vi "Set S34CON wrapper.vi"(7 "bAckEna":i32, 8 "error in (no error)":errorcluster caption="错误输入（无错误）", 9 "S34CON In":T1, 10 "dwCanNodeId":u32, 11 "dwDevIndex":u32) -> (0 "error out":errorcluster caption="错误输出", 1 "S34CON Out":T1, 3 "function return":u32)   [LabVIEW 2016, in "UISimCanFunc_wrapper.lvlib"]
doc: "_declspec (dllexport) DWORD SetS34CON_wrapper(DWORD dwDevIndex, DWORD dwCanNodeId, P_S34CON pS34ConIn, BOOL bAckEna, P_S34CON pS34ConOut);"
uses:
  <userlib>/UISimCanFunc_wrapper/UISimCanFunc_wrapper.lvlib
  <userlib>/UISimCanFunc_wrapper/ctl/S34CON.ctl
  <userlib>/UISimCanFunc_wrapper/UISimCanFunc_wrapper.dll
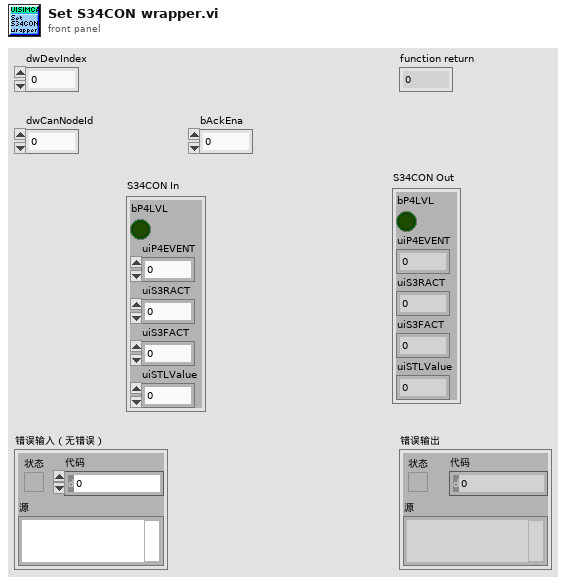
[diagram p1: front panel]
types:
  T1 = typedef "UISimCanFunc_wrapper.lvlib/S34CON.ctl" = cluster{"bP4LVL":bool, "uiP4EVENT":u32, "uiS3RACT":u32, "uiS3FACT":u32, "uiSTLValue":u32}
  T2 = cluster{"bP4LVL":i32, "uiP4EVENT":u32, "uiS3RACT":u32, "uiS3FACT":u32, "uiSTLValue":u32}
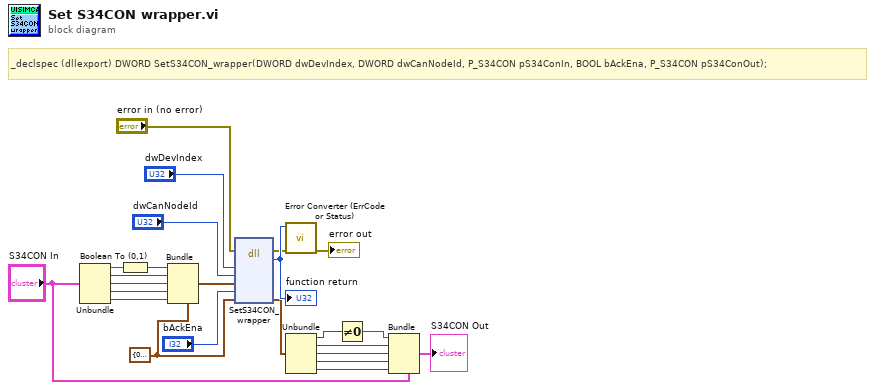
[diagram p0: block diagram]
diagram:
  w10 = T2 {"bP4LVL"=0, "uiP4EVENT"=0, "uiS3RACT"=0, "uiS3FACT"=0, "uiSTLValue"=0} ("pS34ConOut")
  # "_declspec (dllexport) DWORD SetS34CON_wrapper(DWORD dwDevIndex, DWORD dwCanNodeId, P_S34CON pS34ConIn, BOOL bAckEna, P_S34CON pS34ConOut);"
  n1 = Unbundle("S34CON In") -> ("bP4LVL"=w13:bool, "uiP4EVENT"=w17:u32, "uiS3RACT"=w16:u32, "uiS3FACT"=w15:u32, "uiSTLValue"=w14:u32)
  n2 = Boolean To (0,1)(Boolean=w13) -> (0, 1=w12:i16)
  n3 = Bundle(cluster=w10, "bP4LVL"=w12, "uiP4EVENT"=w17, "uiS3RACT"=w16, "uiS3FACT"=w15, "uiSTLValue"=w14) -> (w11:T2)
  n4 = dll-call lib="C:/Program Files (x86)/National Instruments/LabVIEW 2016/user.lib/UISimCanFunc_wrapper/UISimCanFunc_wrapper.*" fn="SetS34CON_wrapper"(error in="error in (no error)", "dwDevIndex"="dwDevIndex", "dwCanNodeId"="dwCanNodeId", "pS34ConIn"=w11, "bAckEna"="bAckEna", "pS34ConOut"=w10) -> (error out=w19:errorcluster, w24:u32, "pS34ConOut"=w9:T2)  [unwired: 6 in, 1 out]
  "function return" <- w24
  n5 = call <userlib>:"Error Converter (ErrCode or Status).vi"("error in (no error)"=w19, "error code"=w24) -> ("error out"=→"error out":errorcluster)  [unwired: 9 in]
  n6 = Unbundle(w9) -> ("bP4LVL"=w3:i32, "uiP4EVENT"=w7:u32, "uiS3RACT"=w6:u32, "uiS3FACT"=w5:u32, "uiSTLValue"=w4:u32)
  n7 = Not Equal To 0?(x=w3) -> (x != 0?=w2:bool)
  n8 = Bundle(cluster="S34CON In", "bP4LVL"=w2, "uiP4EVENT"=w7, "uiS3RACT"=w6, "uiS3FACT"=w5, "uiSTLValue"=w4) -> (→"S34CON Out":T1)
